vi "X10468 SLM Make RT Arrays.vi"(7 "Holo Diameter (px)":i32) -> (4 "R Array":dbl[][](array[numeric]), 8 "Theta Array":dbl[][](array[numeric]), 15 "Mask Array":dbl[][](array[numeric]))   [LabVIEW 2018]
uses:
  <vilib>/Analysis/coordinate.llb/3D Coordinate Conversion (Array).vi
  <vilib>/Analysis/NI_AALPro.lvlib
panel:
  out "Mask":dbl[][](graph)
  out "Theta":dbl[][](graph)
  out "R":dbl[][](graph)
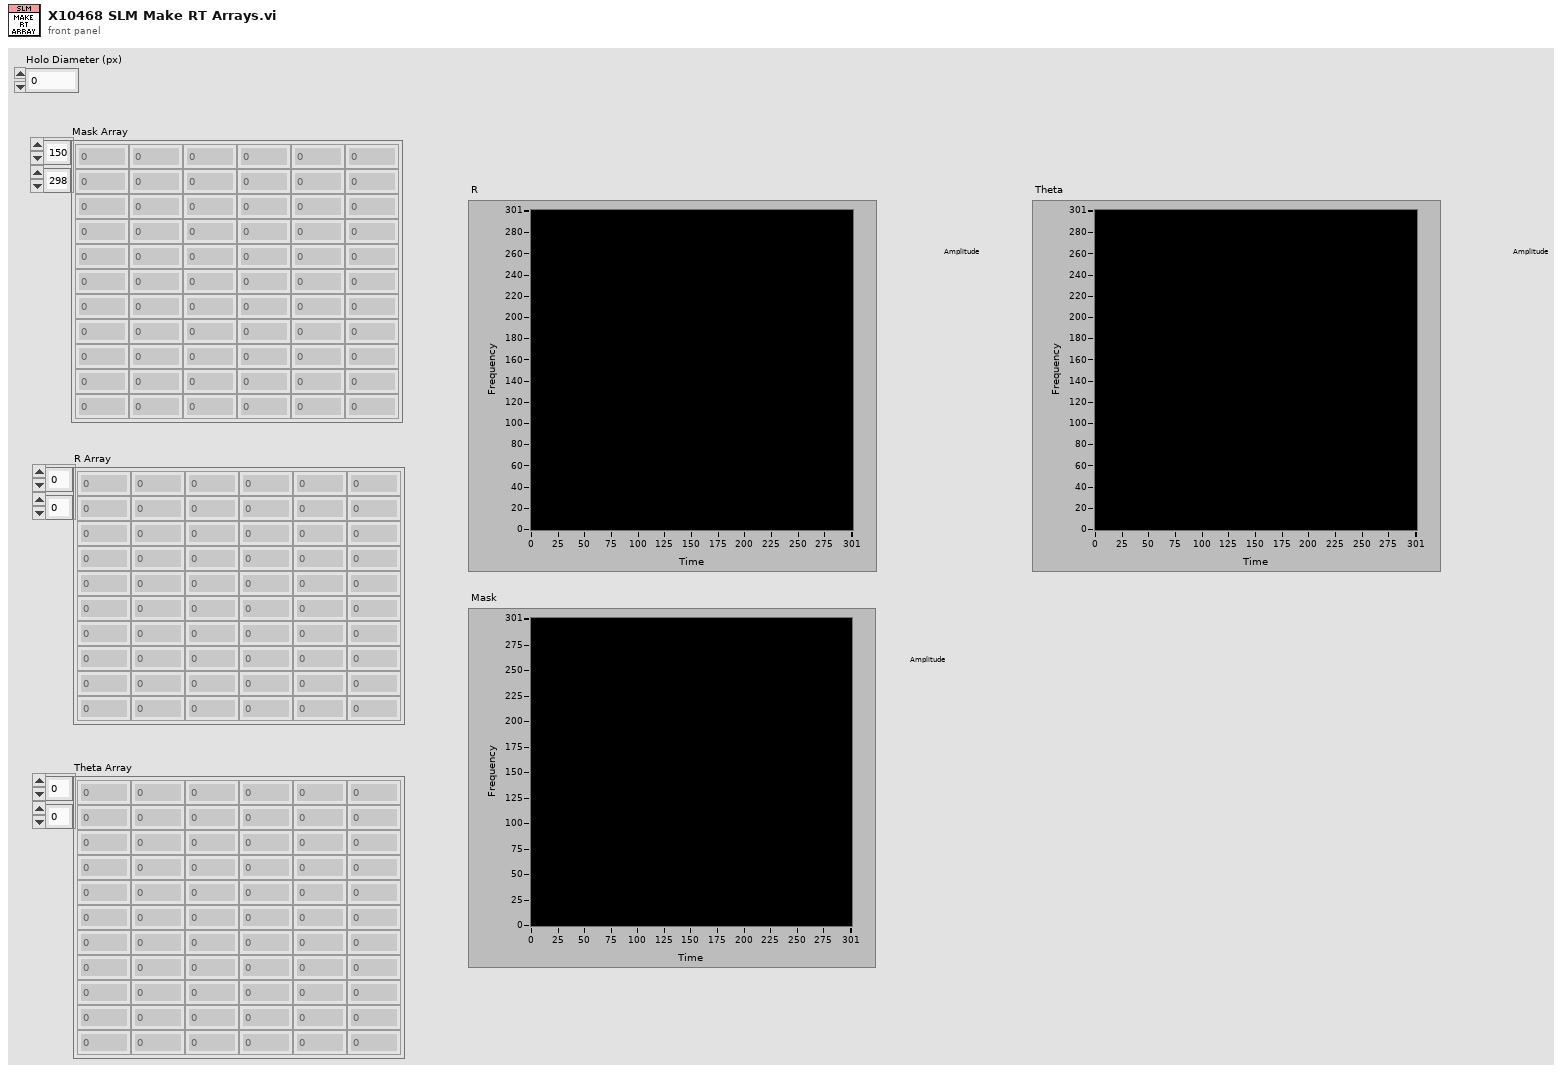
[diagram p1: front panel]
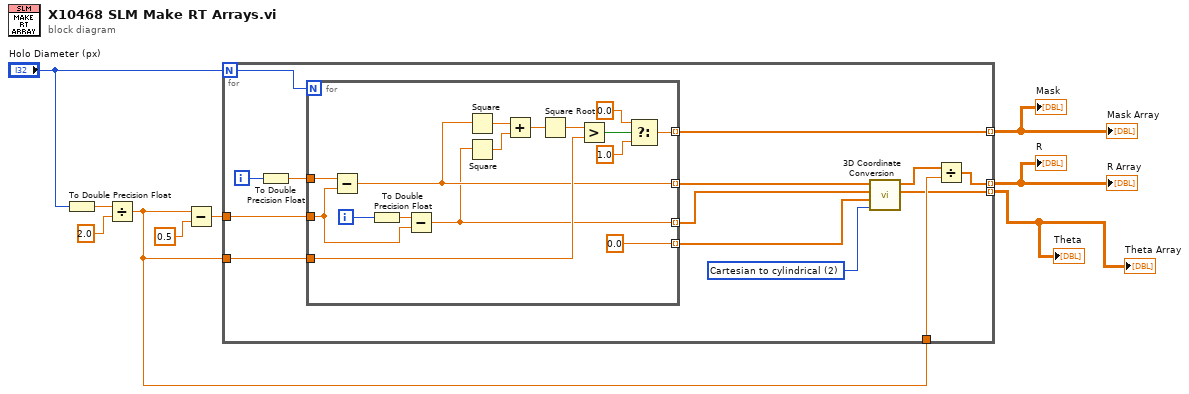
[diagram p0: block diagram]
diagram:
  n1 = To Double Precision Float(number="Holo Diameter (px)") -> (double precision float=w8:dbl)
  n2 = Divide(x=w8, y=2.0) -> (x/y=w1:dbl)
  n3 = Subtract(x=w1, y=0.5 ("Center Correction")) -> (x-y=w6:dbl)
  n4 = for {
    N: "Holo Diameter (px)" -> [w23]
    tunnel: w6 -> [w21]
    tunnel: w1 -> [w20]
    tunnel: [w15] -> w4 mode=indexing
    tunnel: [w10] -> w2 mode=indexing
    tunnel: [w18] -> w3 mode=indexing
    tunnel: w1 -> [w16]
    i -> [w19]
    w12 = u16 2 items=["Cartesian to spherical", "spherical to Cartesian", "Cartesian to cylindrical", "cylindrical to Cartesian", "spherical to cylindrical", "cylindrical to spherical"] ("conversion type")
    n5 = To Double Precision Float(number=w19) -> (double precision float=w22:dbl)
    n6 = for {
      N: w23 -> [_]
      tunnel: w22 -> [w39]
      tunnel: w21 -> [w38]
      tunnel: w20 -> [w30]
      tunnel: [w25] -> w11 mode=indexing
      tunnel: [0.0 ("y")] -> w13 mode=indexing
      tunnel: [w26] -> w18 mode=indexing
      tunnel: [w24] -> w14 mode=indexing
      i -> [w36]
      n7 = Subtract(x=w39, y=w38) -> (x-y=w25:dbl)
      n8 = To Double Precision Float(number=w36) -> (double precision float=w37:dbl)
      n9 = Subtract(x=w37, y=w38) -> (x-y=w24:dbl)
      n10 = Square(x=w25) -> (x^2=w34:dbl)
      n11 = Square(x=w24) -> (x^2=w33:dbl)
      n12 = Add(x=w34, y=w33) -> (x+y=w32:dbl)
      n13 = Square Root(x=w32) -> (sqrt(x)=w31:dbl)
      n14 = Greater?(x=w31, y=w30) -> (0:w29:bool)
      n15 = Select(t=0.0 ("y"), s=w29, f=1.0) -> (s? t:f=w26:dbl)
    }
    n16 = call-poly <vilib>:"3D Coordinate Conversion.vi"("conversion type"=w12, "Axis 3"=w13, "Axis 2"=w14, "Axis 1"=w11) -> ("Axis 2 Out"=w10:dbl[], "Axis 1 Out"=w17:dbl[])  [unwired: 4 in, 2 out]
    n17 = Divide(x=w17, y=w16) -> (x/y=w15:dbl[])
  }
  "Theta Array" <- w2
  "Mask Array" <- w3
  "R Array" <- w4
  "R" <- w4
  "Theta" <- w2
  "Mask" <- w3
